vi "PERFUME.vi"() -> ()   [LabVIEW 2021]
uses:
  <vilib>/numeric/Random Number (Range) U64.vi
  <vilib>/numeric/sub_Random U32.vi
  <vilib>/Utility/file.llb/Write Delimited Spreadsheet (string).vi
  <vilib>/Utility/file.llb/Read Delimited Spreadsheet (string).vi
panel:
  out "EVENTS":string[][](array[string])
  out "CURRENT CLUSTER":T1
  out "DATA FILE ERROR IF ANY":errorcluster
  out "NUMBER OF JASMINE PERFUME":dbl
  out "NUMBER OF ROSE PERFUME":dbl
  out "NUMBER OF LAVENDAR PERFUME":dbl
  out "NUMBER OF BERGAMOT PERFUME":dbl
  out "TOTAL NUMBER OF EVENT":dbl
  out "CURRENT EVENT":string
  out "ETHANOL PRICE":dbl
  out "BUS":dbl(slide) scale=0.0..10.0
  out "Packaging":dbl(slide) scale=0.0..10.0
  out "MIXTURE":u8(slide)
  out "StOIL":u8(slide) scale=0.0..10.0
  out "StCo2":u8(slide)
  out "PRESSURE":dbl(knob) scale=0.0..130.0
  out "SEPERATOR":dbl(slide) scale=0.0..10.0
  out "PRV2":u8(slide) scale=0.0..10.0
  out "PRV":u8(slide) scale=0.0..10.0
  out "PRV1":u8(slide) scale=0.0..10.0
  out "RAW TO CO2":u8(slide) scale=0.0..10.0
  out "RAW TO CO2":u8(slide) scale=0.0..10.0
  out "Co2 Tank":dbl(slide)
  out "MATERIAL TANK":dbl(slide) scale=0.0..10.0
  out "FLOWER TANK":u8(slide) scale=0.0..10.0
  out "JASMINE":bool
  out "ROSE":bool
  out "LAVENDAR":bool
  out "BERGAMOT":bool
  out "LAVENDAR TANK":dbl(slide) scale=0.0..10.0
  out "BERGAMOT TANK":dbl(slide) scale=0.0..10.0
  out "JASMINE TANK":dbl(slide) scale=0.0..10.0
  out "ROSE TANK":dbl(slide) scale=0.0..10.0
  out "WATER":dbl(slide)
  out "AROMA":dbl(slide)
  out "LIQUOR":dbl(slide)
  out "OIL":dbl(slide)
  out "SELECTED TYPE":string
  out "Thermometer":dbl(slide) scale=0.0..120.0
  # "RAW MATERIALS SYSTEM"
  # "CO2 EXTRACTION"
  # "MIXING"
  # "PACKAGING"
  # "Maintain temperature between 95 to 100"
  # "Co2 brough back to natural pressure"
  # "PUMP"
  # "PRESSURE REDUCING VALVE"
  # "Dispatch"
  # "INFORMATION PANEL"
  # "USD"
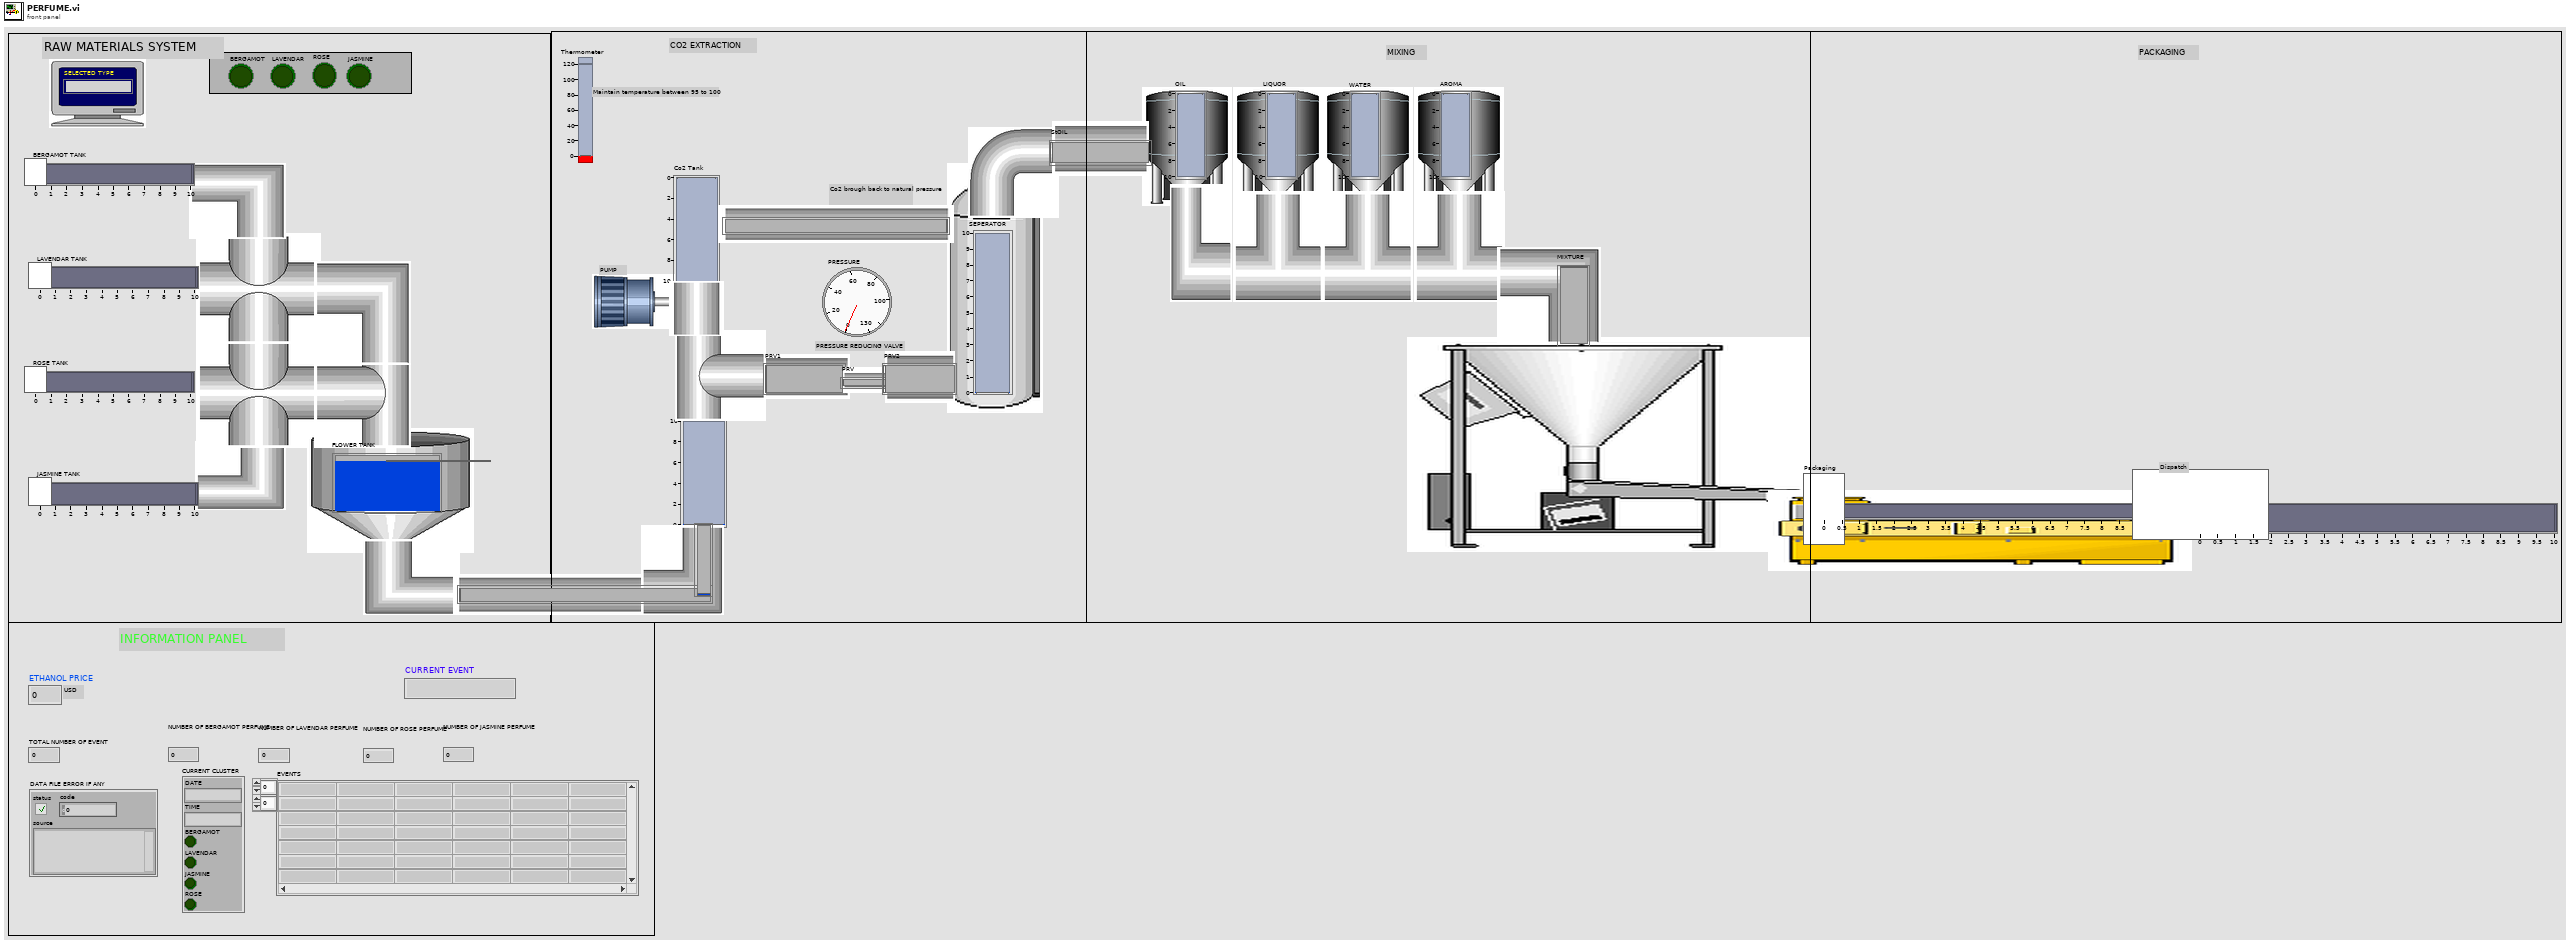
[diagram p1: front panel]
types:
  T1 = cluster{"DATE":string, "TIME":string, "BERGAMOT":bool, "LAVENDAR":bool, "JASMINE":bool, "ROSE":bool}
  T2 = cluster{"date string":string, "time string":string, "BERGAMOT":bool, "LAVENDAR":bool, "JASMINE":bool, "ROSE":bool}
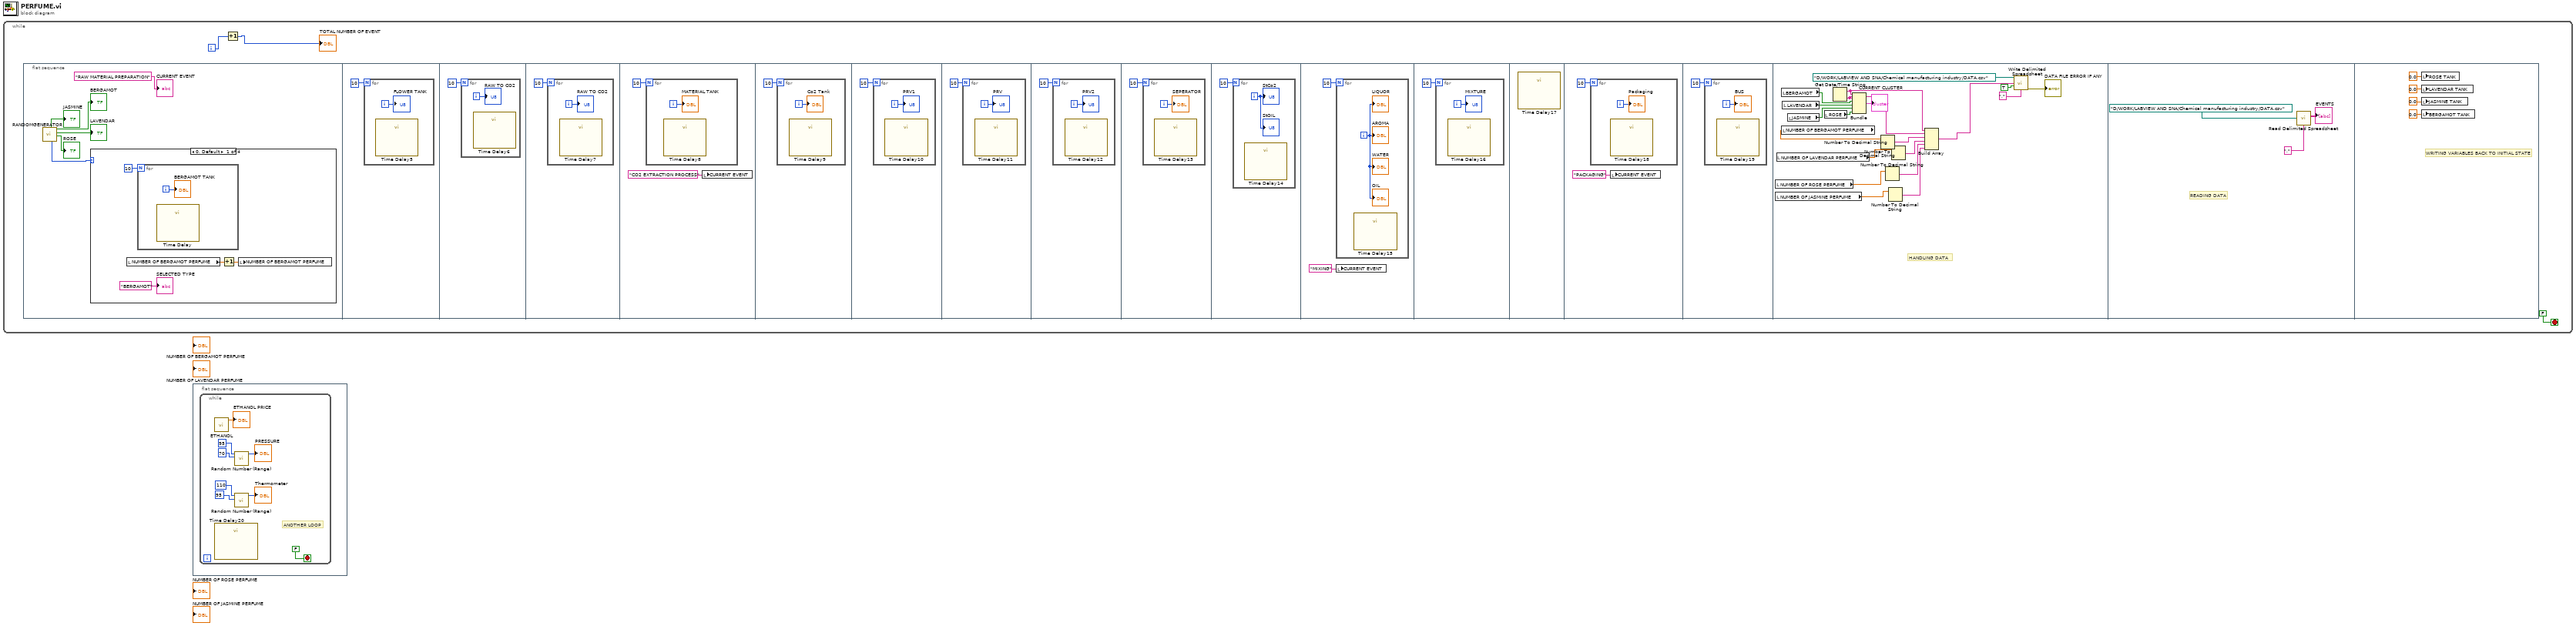
[diagram p0: block diagram]
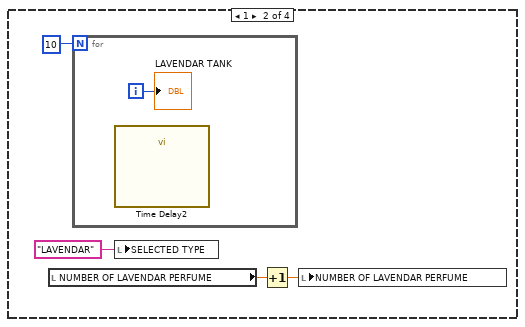
[diagram p2: hidden frame]
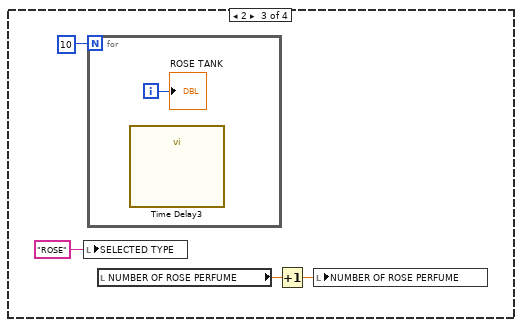
[diagram p3: hidden frame]
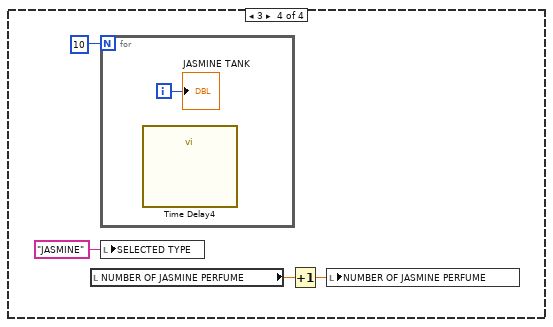
[diagram p4: hidden frame]
diagram:
  n1 = while {
    i -> [w2]
    stop <- FALSE stop-if-true
    n2 = flat-sequence {
      frame #0 {
        n3 = call "RANDOMGENERATOR.vi"() -> ("Boolean 4"=→"ROSE":bool, "Boolean 2"=→"LAVENDAR":bool, "Boolean 3"=→"BERGAMOT":bool, "index of element"=w5:i32, "Boolean"=→"JASMINE":bool)  [unwired: 7 in]
        n4 = case shown="0, Default" w5 {
          frame 0, Default {
            n5 = local read "NUMBER OF BERGAMOT PERFUME"() -> (w11:dbl)
            n6 = for {
              N: 10 -> [_]
              i -> [w14]
              n7 = call "Time Delay"() -> ()  [unwired: 11 in, 1 out]
              "BERGAMOT TANK" <- w14
            }
            n8 = Increment(x=w11) -> (x+1=w10:dbl)
            n9 = local write "NUMBER OF BERGAMOT PERFUME"(w10) -> ()
            "SELECTED TYPE" <- "BERGAMOT" ("SELECTED TYPE")
          }
          frame 1 {
            n10 = local read "NUMBER OF LAVENDAR PERFUME"() -> (w15:dbl)
            n11 = for {
              N: 10 -> [_]
              i -> [w19]
              n12 = call "Time Delay2"() -> ()  [unwired: 11 in, 1 out]
              "LAVENDAR TANK" <- w19
            }
            n13 = local write "SELECTED TYPE"("LAVENDAR" ("SELECTED TYPE")) -> ()
            n14 = Increment(x=w15) -> (x+1=w16:dbl)
            n15 = local write "NUMBER OF LAVENDAR PERFUME"(w16) -> ()
          }
          frame 2 {
            n16 = local write "SELECTED TYPE"("ROSE" ("SELECTED TYPE")) -> ()
            n17 = for {
              N: 10 -> [_]
              i -> [w24]
              n18 = call "Time Delay3"() -> ()  [unwired: 11 in, 1 out]
              "ROSE TANK" <- w24
            }
            n19 = local read "NUMBER OF ROSE PERFUME"() -> (w20:dbl)
            n20 = Increment(x=w20) -> (x+1=w21:dbl)
            n21 = local write "NUMBER OF ROSE PERFUME"(w21) -> ()
          }
          frame 3 {
            n22 = local read "NUMBER OF JASMINE PERFUME"() -> (w25:dbl)
            n23 = for {
              N: 10 -> [_]
              i -> [w29]
              n24 = call "Time Delay4"() -> ()  [unwired: 11 in, 1 out]
              "JASMINE TANK" <- w29
            }
            n25 = local write "SELECTED TYPE"("JASMINE" ("SELECTED TYPE")) -> ()
            n26 = Increment(x=w25) -> (x+1=w26:dbl)
            n27 = local write "NUMBER OF JASMINE PERFUME"(w26) -> ()
          }
        }
        "CURRENT EVENT" <- "RAW MATERIAL PREPARATION" ("CURRENT EVENT")
      }
      frame #1 {
        n28 = for {
          N: 10 -> [_]
          i -> [w31]
          n29 = call "Time Delay5"() -> ()  [unwired: 11 in, 1 out]
          "FLOWER TANK" <- w31
        }
      }
      frame #2 {
        n30 = for {
          N: 10 -> [_]
          i -> [w33]
          n31 = call "Time Delay6"() -> ()  [unwired: 11 in, 1 out]
          "RAW TO CO2" <- w33
        }
      }
      frame #3 {
        n32 = for {
          N: 10 -> [_]
          i -> [w35]
          n33 = call "Time Delay7"() -> ()  [unwired: 11 in, 1 out]
          "RAW TO CO2" <- w35
        }
      }
      frame #4 {
        n34 = for {
          N: 10 -> [_]
          i -> [w38]
          n35 = call "Time Delay8"() -> ()  [unwired: 11 in, 1 out]
          "MATERIAL TANK" <- w38
        }
        n36 = local write "CURRENT EVENT"("CO2 EXTRACTION PROCESS" ("CURRENT EVENT")) -> ()
      }
      frame #5 {
        n37 = for {
          N: 10 -> [_]
          i -> [w40]
          n38 = call "Time Delay9"() -> ()  [unwired: 11 in, 1 out]
          "Co2 Tank" <- w40
        }
      }
      frame #6 {
        n39 = for {
          N: 10 -> [_]
          i -> [w42]
          n40 = call "Time Delay10"() -> ()  [unwired: 11 in, 1 out]
          "PRV1" <- w42
        }
      }
      frame #7 {
        n41 = for {
          N: 10 -> [_]
          i -> [w44]
          n42 = call "Time Delay11"() -> ()  [unwired: 11 in, 1 out]
          "PRV" <- w44
        }
      }
      frame #8 {
        n43 = for {
          N: 10 -> [_]
          i -> [w46]
          n44 = call "Time Delay12"() -> ()  [unwired: 11 in, 1 out]
          "PRV2" <- w46
        }
      }
      frame #9 {
        n45 = for {
          N: 10 -> [_]
          i -> [w48]
          n46 = call "Time Delay13"() -> ()  [unwired: 11 in, 1 out]
          "SEPERATOR" <- w48
        }
      }
      frame #10 {
        n47 = for {
          N: 10 -> [_]
          i -> [w50]
          n48 = call "Time Delay14"() -> ()  [unwired: 11 in, 1 out]
          "StCo2" <- w50
          "StOIL" <- w50
        }
      }
      frame #11 {
        n49 = for {
          N: 10 -> [_]
          i -> [w53]
          n50 = call "Time Delay15"() -> ()  [unwired: 11 in, 1 out]
          "OIL" <- w53
          "LIQUOR" <- w53
          "AROMA" <- w53
          "WATER" <- w53
        }
        n51 = local write "CURRENT EVENT"("MIXING" ("CURRENT EVENT")) -> ()
      }
      frame #12 {
        n52 = for {
          N: 10 -> [_]
          i -> [w55]
          n53 = call "Time Delay16"() -> ()  [unwired: 11 in, 1 out]
          "MIXTURE" <- w55
        }
      }
      frame #13 {
        n54 = call "Time Delay17"() -> ()  [unwired: 11 in, 1 out]
      }
      frame #14 {
        n55 = for {
          N: 10 -> [_]
          i -> [w58]
          n56 = call "Time Delay18"() -> ()  [unwired: 11 in, 1 out]
          "Packaging" <- w58
        }
        n57 = local write "CURRENT EVENT"("PACKAGING" ("CURRENT EVENT")) -> ()
      }
      frame #15 {
        n58 = for {
          N: 10 -> [_]
          i -> [w60]
          n59 = call "Time Delay19"() -> ()  [unwired: 11 in, 1 out]
          "BUS" <- w60
        }
      }
      frame #16 {
        # "HANDLING DATA"
        n60 = local read "NUMBER OF ROSE PERFUME"() -> (w65:dbl)
        n61 = local read "NUMBER OF JASMINE PERFUME"() -> (w63:dbl)
        n62 = local read "NUMBER OF LAVENDAR PERFUME"() -> (w67:dbl)
        n63 = local read "BERGAMOT"() -> (w76:bool)
        n64 = local read "NUMBER OF BERGAMOT PERFUME"() -> (w71:dbl)
        n65 = local read "LAVENDAR"() -> (w74:bool)
        n66 = local read "JASMINE"() -> (w75:bool)
        n67 = local read "ROSE"() -> (w73:bool)
        n68 = Get Date/Time String() -> (date string=w70:string, time string=w69:string)  [unwired: 3 in]
        n69 = Bundle("date string"=w70, "time string"=w69, "BERGAMOT"=w76, "LAVENDAR"=w74, "JASMINE"=w75, "ROSE"=w73) -> (→"CURRENT CLUSTER":T2)  [unwired: 1 in]
        n70 = Number To Decimal String(number=w71) -> (decimal integer string=w68:string)  [unwired: 1 in]
        n71 = Number To Decimal String(number=w65) -> (decimal integer string=w64:string)  [unwired: 1 in]
        n72 = Number To Decimal String(number=w63) -> (decimal integer string=w62:string)  [unwired: 1 in]
        n73 = Number To Decimal String(number=w67) -> (decimal integer string=w66:string)  [unwired: 1 in]
        n74 = Build Array(w70, w69, w68, w66, w64, w62) -> (w61:string[])
        n75 = call-poly <vilib>:"Write Delimited Spreadsheet.vi"("file path (dialog if empty)"=path "D:/WORK/LABVIEW AND SNA/Chemical manufacturing industry/DATA.csv", "1D data"=w61, "append to file? (new file:F)"=TRUE, "delimiter (\\t)"="," ("delimiter (\\t)")) -> ("error out"=→"DATA FILE ERROR IF ANY":errorcluster)  [unwired: 10 in, 1 out]
      }
      frame #17 {
        # "READING DATA"
        n76 = call-poly <vilib>:"Read Delimited Spreadsheet.vi"("file path (dialog if empty)"=path "D:/WORK/LABVIEW AND SNA/Chemical manufacturing industry/DATA.csv", "delimiter (\\t)"="," ("delimiter (\\t)")) -> ("all rows"=→"EVENTS":string[][])  [unwired: 8 in, 5 out]
      }
      frame #18 {
        # "WRITING VARIABLES BACK TO INITIAL STATE"
        n77 = local write "ROSE TANK"(0.0 ("ROSE TANK")) -> ()
        n78 = local write "LAVENDAR TANK"(0.0 ("LAVENDAR TANK")) -> ()
        n79 = local write "JASMINE TANK"(0.0 ("JASMINE TANK")) -> ()
        n80 = local write "BERGAMOT TANK"(0.0 ("BERGAMOT TANK")) -> ()
      }
    }
    n81 = Increment(x=w2) -> (x+1=→"TOTAL NUMBER OF EVENT":i32)
  }
  n82 = flat-sequence {
    frame #0 {
      n83 = while {
        stop <- FALSE stop-if-true
        # "ANOTHER LOOP"
        n84 = call "ETHANOL.vi"() -> ("Numeric"=→"ETHANOL PRICE":dbl)  [unwired: 11 in]
        n85 = call "Time Delay20"() -> ()  [unwired: 11 in, 1 out]
        n86 = call-poly <vilib>:"Random Number (Range).vi"("lower bound (0)"=u64 70, "upper bound (100)"=u64 95) -> ("number"=→"PRESSURE":u64)  [unwired: 9 in]
        n87 = call-poly <vilib>:"Random Number (Range).vi"("lower bound (0)"=u64 95, "upper bound (100)"=u64 110) -> ("number"=→"Thermometer":u64)  [unwired: 9 in]
      }
    }
  }
